vi "SwerveOrientationLock.vi"(0 "Joystick X":dbl, 1 "Joystick Y":dbl, 3 "Joystick Rotation":dbl, 6 "PID Tuning Parameters":T2={"Kp"=0.0, "Ki"=0.0, "Kd"=0.0, "N-Diff"=10, "N-Int"=10, "Int Error Window"=30.0, "Max Ouput"=1.0, "Min Output"=-1.0} {"Int Error Window" min=0.0; "N-Int" min=2; "N-Diff" min=2; "Kd" min=0.0; "Ki" min=0.0; "Kp" min=0.0}, 7 "Rotation Deadband":dbl, 8 "Orientation Lock Delay (ms)":u32, 10 "Orientation Lock Strafe Deadband":dbl, 12 "External Disables":bool) -> (14 "Controller Summary":T1(graph), 17 "Joystick Rotation":dbl, 19 "Auto Rotation Control":bool)   [LabVIEW 2019]
uses:
  sensors.vi
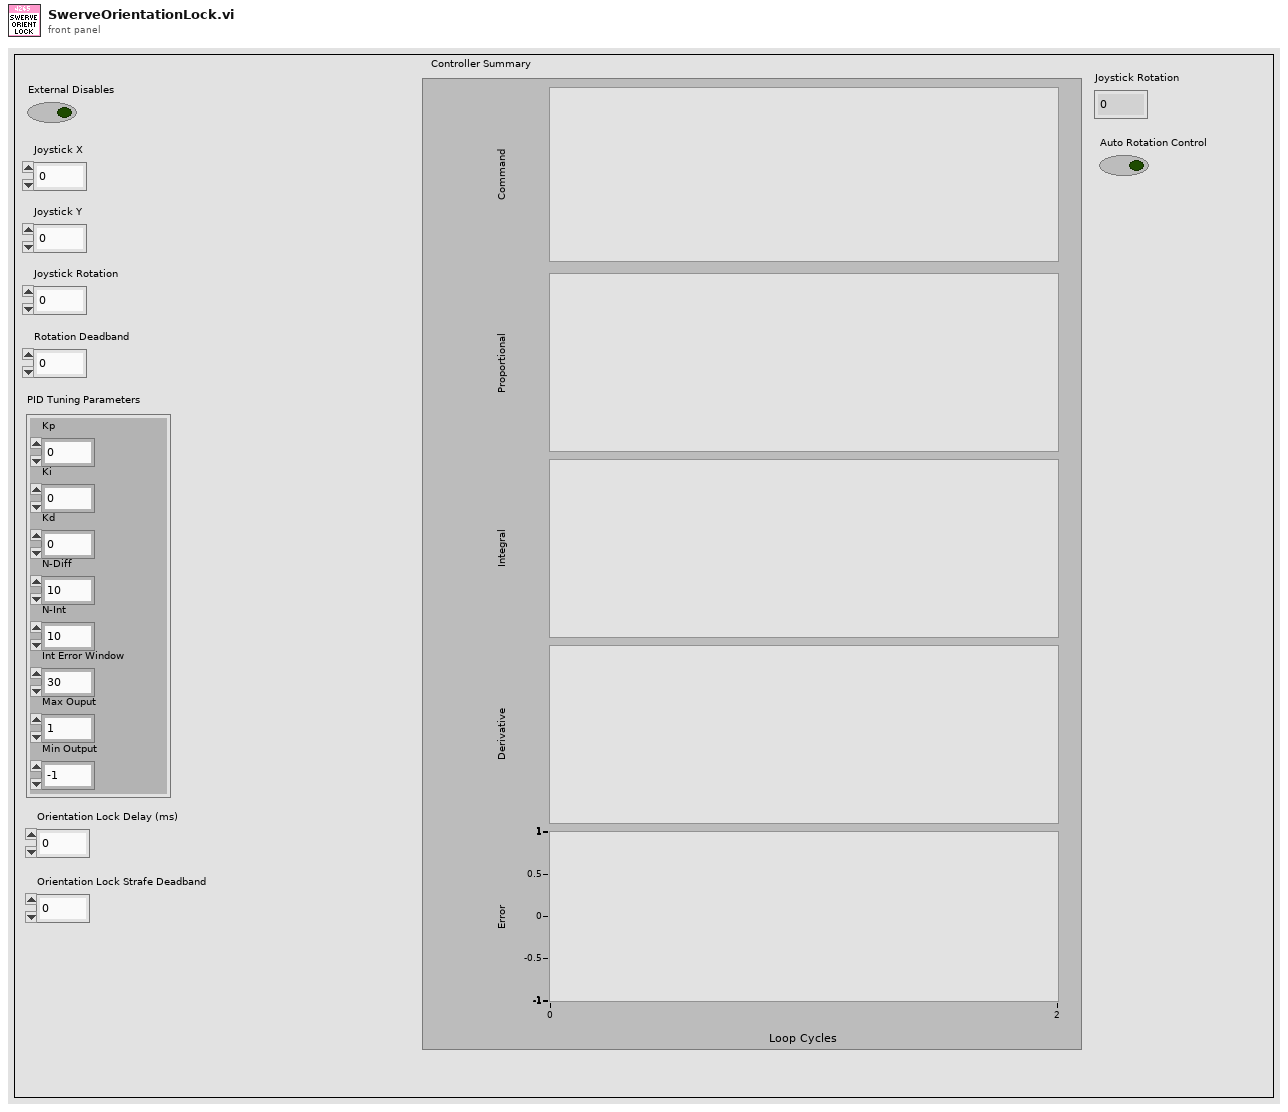
[diagram p1: front panel]
types:
  T1 = cluster{"Command":dbl, "Proportional":dbl, "Integral":dbl, "Derivative":dbl, "Goal":dbl}
  T2 = cluster{"Kp":dbl, "Ki":dbl, "Kd":dbl, "N-Diff":i32, "N-Int":i32, "Int Error Window":dbl, "Max Ouput":dbl, "Min Output":dbl}
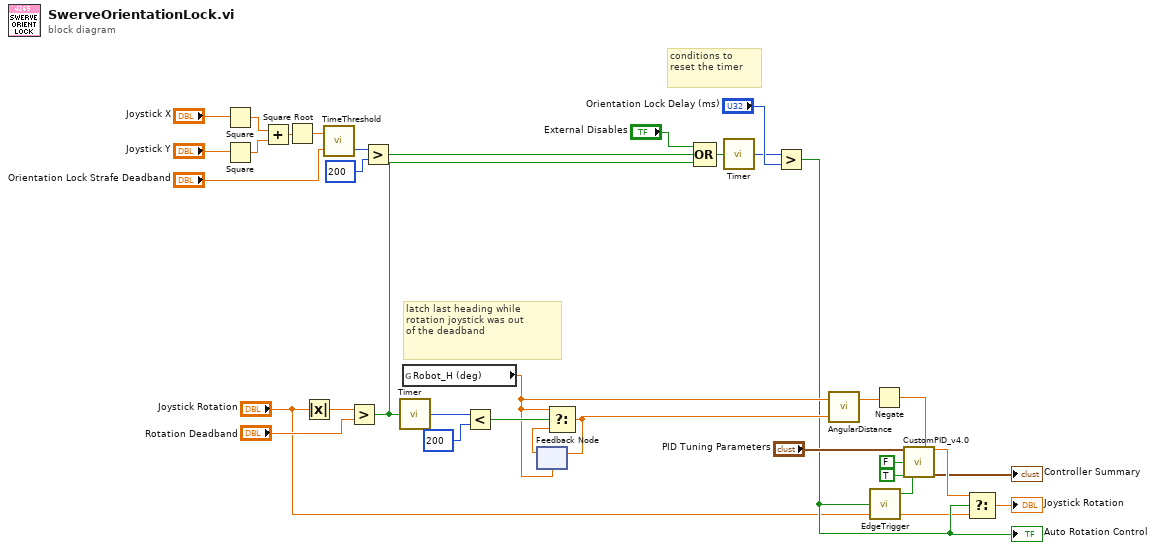
[diagram p0: block diagram]
diagram:
  # "conditions to\nreset the timer"
  # "latch last heading while\nrotation joystick was out \nof the deadband"
  n1 = Square(x="Joystick X") -> (x^2=w12:dbl)
  n2 = Square(x="Joystick Y") -> (x^2=w13:dbl)
  n3 = Add(x=w12, y=w13) -> (x+y=w11:dbl)
  n4 = Square Root(x=w11) -> (sqrt(x)=w30:dbl)
  n5 = Absolute Value(x="Joystick Rotation") -> (abs(x)=w10:dbl)
  n6 = call "TimeThreshold.vi"("Threshold"="Orientation Lock Strafe Deadband", "Current Value"=w30) -> ("Time Below Threshold (ms)"=w32:u32)  [unwired: 1 out]
  n7 = Greater?(x=w10, y="Rotation Deadband") -> (0:w27:bool)
  n8 = Greater?(x=w32, y=u32 200) -> (0:w34:bool)
  n9 = call "Timer.vi"("Reset Timer"=w27) -> ("Time (ms)"=w26:u32)
  n10 = global read "sensors.vi" "Robot_H (deg)"() -> (w14:dbl)
  n11 = Less?(x=w26, y=u32 200) -> (x < y?=w29:bool)
  n12 = feedback #1(w14) -> (w16:dbl)
  n13 = Select(t=w14, s=w29, f=w16) -> (s? t:f=w15:dbl)
  n14 = feedback-in #1(w15) -> ()
  n15 = Compound Arithmetic op=OR("External Disables", w34, w27) -> (w7:bool)
  n16 = call "Timer.vi"("Reset Timer"=w7) -> ("Time (ms)"=w8:u32)
  n17 = Greater?(x=w8, y="Orientation Lock Delay (ms)") -> (0:w5:bool)
  "Auto Rotation Control" <- w5
  n18 = call "AngularDistance.vi"("Goal Angle (deg) [0,360]"=w15, "Current Angle (deg) [-Inf,+Inf]"=w14) -> ("Signed Angular Distance (deg) [-180,+180]"=w9:dbl)  [unwired: 1 out]
  n19 = call "EdgeTrigger.vi"("Input Signal"=w5) -> ("Rising Edge Trigger"=w23:bool)  [unwired: 2 out]
  n20 = Negate(x=w9) -> (-x=w21:dbl)
  n21 = call "CustomPID_v4.0.vi"("PID Tuning Parameters"="PID Tuning Parameters", "Custom Error Calculation"=w21, "Reset on Goal Change ?"=FALSE, "Use Custom Error Calculation ?"=TRUE, "Reinit"=w23) -> ("Command"=w6:dbl, "Controller Summary"=→"Controller Summary":T1)  [unwired: 7 in, 2 out]
  n22 = Select(t=w6, s=w5, f="Joystick Rotation") -> (s? t:f=→"Joystick Rotation":dbl)
